vi "Create Gradient Picture.vi"(7 "Border Settings":T1={"Border"=enum."No Border", "Border Color"=10405366, "Border Width"=2, "Oval Width"=15, "Oval Height"=15}, 8 "Offset":cluster{"x":i16, "y":i16}, 9 "Width":i32=50, 10 "Height":i32=200, 11 "Color Array":u32[](array[colorbox])=[9144575, 11917531, 11534591]) -> (3 "Gradient Picture":picture)   [LabVIEW 2016, in "Graphics.lvclass"]
doc: "This VI will draw a gradient picture, which is a 2D picture that is a rectangle at the specified offset, with the height and width provided. Drawing the borders will make the rectangle or rounded rectangle with a border color selected. The gradient goes from the Color Array where index 0 is the top and the last element is the bottom with a gradient between.\n\nhttps://decibel.ni.com/content/docs/DOC-9294\n\n-----\nBrian Hoover (hooovahh)"
uses:
  <resource>/Framework/Providers/Open_GDS/UML/Graphics_class/Graphics.lvclass
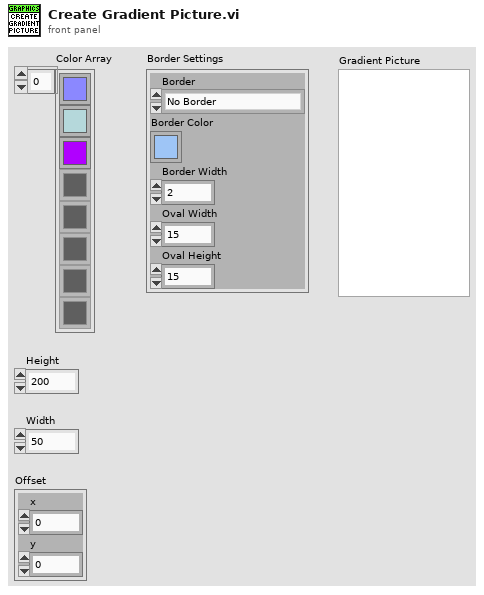
[diagram p1: front panel]
types:
  T1 = cluster{"Border":enum16{"No Border", "Rectangle", "Rounded Rectangle"}, "Border Color":u32, "Border Width":i16, "Oval Width":i16, "Oval Height":i16}
  T2 = enum16{"No Border", "Rectangle", "Rounded Rectangle"}
  T3 = cluster{"left":i16, "top":i16, "right":i16, "bottom":i16}
  T4 = cluster{"Width":i16, "Style":enum32{"Solid", "Dash", "Dot", "DashDot", "DashDotDot"}}
  T5 = cluster{"Width":u16, "Style":enum32{"Solid", "Dash", "Dot", "DashDot", "DashDotDot"}}
  T6 = cluster{"Height":i32, "Width":i32, "Oval Height":i16, "Oval Height":i16, "Border":enum16{"No Border", "Rectangle", "Rounded Rectangle"}, "Border Width":i16, "Border Color":u32}
  T7 = typedef "imagedata.ctl" = cluster{"image type":i32, "image depth":i32, "image":u8[], "mask":u8[], "colors":u32[], "Rectangle":cluster{"left":i16, "top":i16, "right":i16, "bottom":i16}}
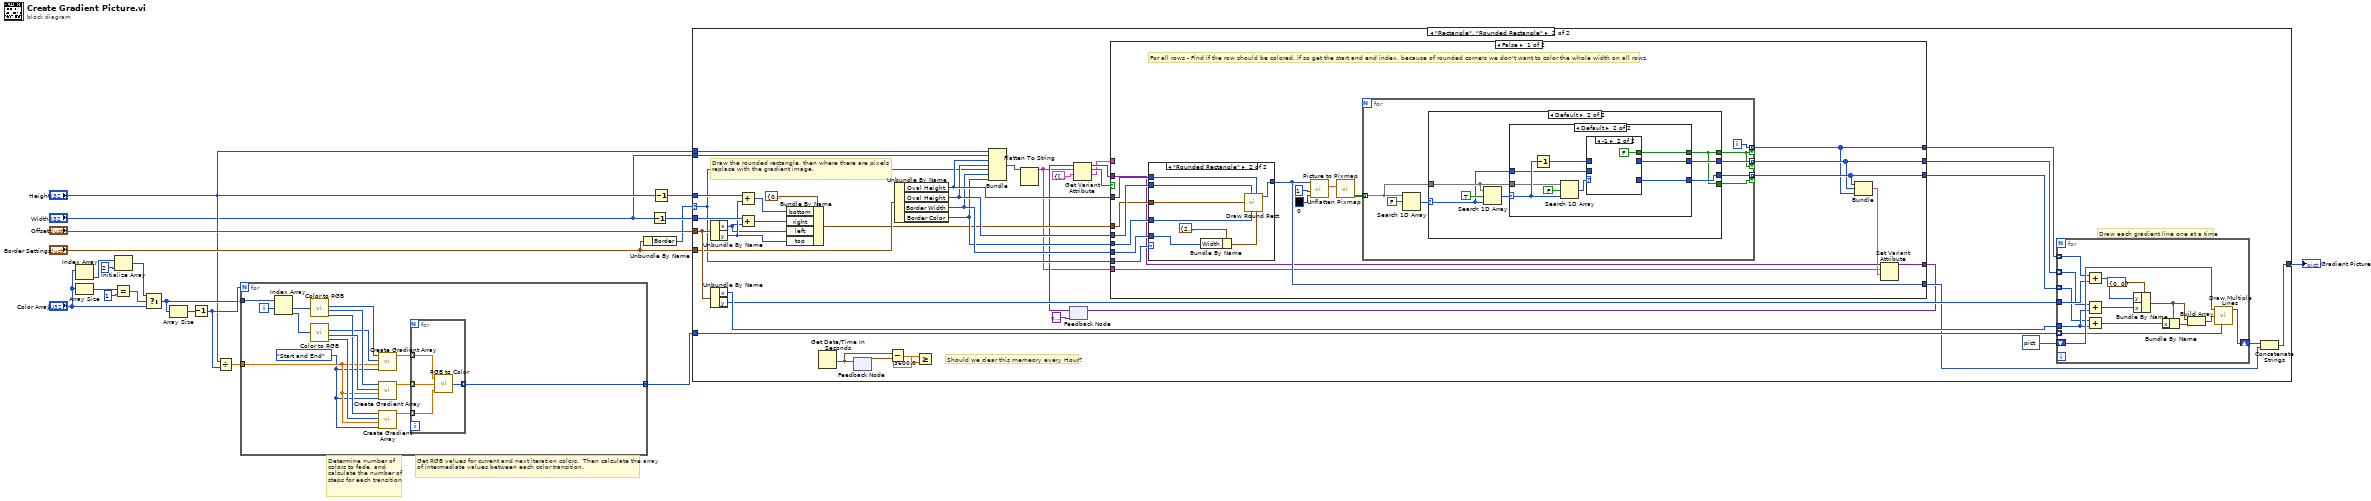
[diagram p0: block diagram]
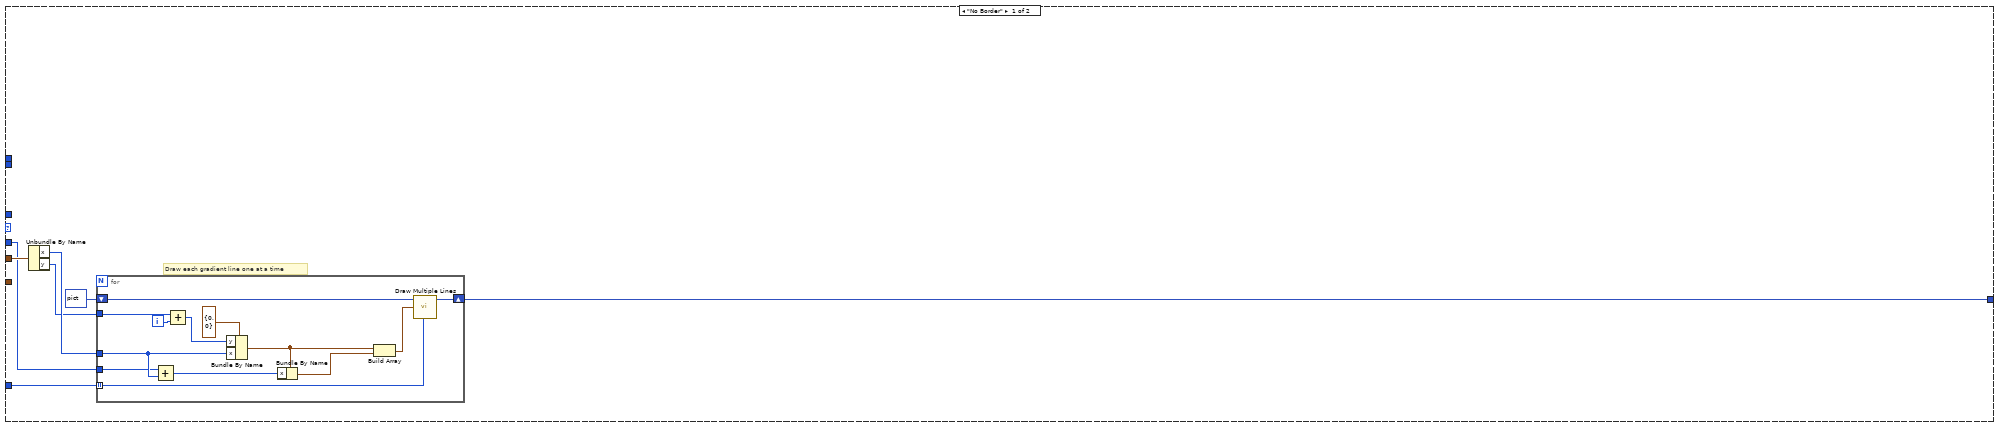
[diagram p2: hidden frame]
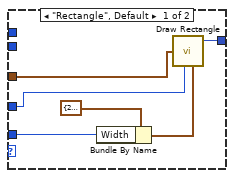
[diagram p3: hidden frame]
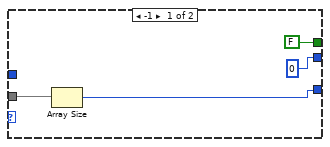
[diagram p5: hidden frame]
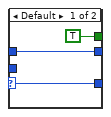
[diagram p6: hidden frame]
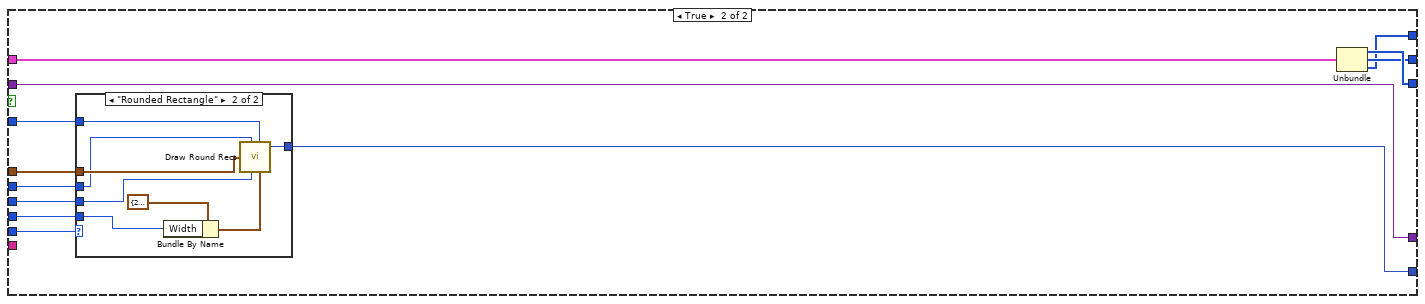
[diagram p7: hidden frame]
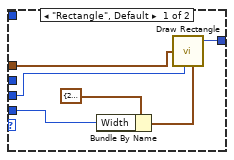
[diagram p8: hidden frame]
diagram:
  # "Get RGB values for current and next iteration colors.  Then calculate the array of intermediate values between each color transition."
  # "Determine number of colors to fade, and calculate the number of steps for each transition"
  n1 = Index Array(array="Color Array") -> (element=w8:u32)  [unwired: 1 in]
  n2 = Array Size(array="Color Array") -> (size(s)=w12:i32)
  n3 = Equal?(x=w12, y=1) -> (x = y?=w10:bool)
  n4 = Initialize Array(w8, 2 ("dimension size")) -> (w6:u32[])
  n5 = Select(t=w6, s=w10, f="Color Array") -> (s? t:f=w5:u32[])
  n6 = Array Size(array=w5) -> (size(s)=w19:i32)
  n7 = Decrement(x=w19) -> (x-1=w18:i32)
  n8 = Divide(x="Height", y=w18) -> (x/y=w20:dbl)
  n9 = for {
    N: w18 -> [_]
    tunnel: w5 -> [w36]
    tunnel: w20 -> [w27]
    tunnel: [w22] -> w17 mode=concatenating
    i -> [w35]
    w26 = enum16{"Start", "End", "Start and End", "None"}."Start and End" ("Values to Include")
    n10 = Index Array(array=w36, index #1=w35) -> (element #1=w34:u32, element #2=w33:u32)  [unwired: 1 in]
    n11 = call <vilib>:"Color to RGB.vi"("Color"=w34) -> ("R"=w32:u8, "G"=w31:u8, "B"=w29:u8)  [unwired: 1 out]
    n12 = call <vilib>:"Color to RGB.vi"("Color"=w33) -> ("R"=w21:u8, "G"=w30:u8, "B"=w28:u8)  [unwired: 1 out]
    n13 = call <resource>:"Create Gradient Array.vi"("Values to Include"=w26, "Array Length"=w27, "End Value"=w21, "Start Value"=w32) -> ("Output Array"=w25:dbl[])  [unwired: 7 in]
    n14 = call <resource>:"Create Gradient Array.vi"("Values to Include"=w26, "Array Length"=w27, "End Value"=w30, "Start Value"=w31) -> ("Output Array"=w24:dbl[])  [unwired: 7 in]
    n15 = call <resource>:"Create Gradient Array.vi"("Values to Include"=w26, "Array Length"=w27, "End Value"=w28, "Start Value"=w29) -> ("Output Array"=w23:dbl[])  [unwired: 7 in]
    n16 = for {
      tunnel: w25 -> [w39] mode=indexing
      tunnel: w24 -> [w40] mode=indexing
      tunnel: w23 -> [w38] mode=indexing
      tunnel: [w37] -> w22 mode=indexing
      n17 = call <vilib>:"RGB to Color.vi"("B"=w38, "G"=w40, "R"=w39) -> ("Color"=w37:u32)
    }
  }
  n18 = Unbundle By Name("Border Settings") -> ("Border"=w3:T2)
  n19 = Decrement(x="Width") -> (x-1=w14:i32)
  n20 = Decrement(x="Height") -> (x-1=w15:i32)
  n21 = case shown="\"Rectangle\", \"Rounded Rectangle\"" w3 {
    selector: w3 -> [_ w80]
    tunnel: [w42 w94] -> w13
    tunnel: w17 -> [w43 w92]
    tunnel: "Offset" -> [w44 w91]
    tunnel: w15 -> [_ w90]
    tunnel: w14 -> [w41 w89]
    tunnel: "Border Settings" -> [_ w83]
    tunnel: "Height" -> [_ w66]
    tunnel: "Width" -> [_ w65]
    frame "No Border" {
      # "Draw each gradient line one at a time"
      n22 = Unbundle By Name(w44) -> ("x"=w46:i16, "y"=w45:i16)
      n23 = for {
        shift-right: [w59] -> w42
        shift-left: picture data[5B] ("picture") -> [w60]
        tunnel: w43 -> [w52] mode=indexing
        tunnel: w45 -> [w51]
        tunnel: w46 -> [w54]
        tunnel: w41 -> [w50]
        i -> [w48]
        n24 = Add(x=w50, y=w54) -> (x+y=w53:i32)
        n25 = Add(x=w51, y=w48) -> (x+y=w49:i32)
        n26 = Bundle By Name(cluster=cluster{"x":i16, "y":i16} {"x"=0, "y"=0} ("point(x,y)"), "y"=w49, "x"=w54) -> (w58:cluster{"x":i16, "y":i16})
        n27 = Bundle By Name(cluster=w58, "x"=w53) -> (w57:cluster{"x":i16, "y":i16})
        n28 = Build Array(w58, w57) -> (w56:cluster{"x":i16, "y":i16}[])
        n29 = call <vilib>:"Draw Multiple Lines.vi"("picture"=w60, "line endpoints"=w56, "color(black)"=w52) -> ("new picture"=w59:picture)  [unwired: 6 in]
      }
    }
    frame "Rectangle", "Rounded Rectangle" {
      # "Should we clear this memeory every Hour?"
      # "Draw each gradient line one at a time"
      # "Draw the rounded rectangle, then where there are pixels replace with the gradient image."
      n30 = Unbundle By Name(w91) -> ("x"=w85:i16, "y"=w87:i16)
      n31 = Unbundle By Name(w91) -> ("x"=w98:i16, "y"=w93:i16)
      n32 = Add(x=w90, y=w87) -> (x+y=w86:i32)
      n33 = Add(x=w89, y=w85) -> (x+y=w84:i32)
      n34 = Bundle By Name(cluster=T3 {"left"=0, "top"=0, "right"=0, "bottom"=0} ("rect"), "bottom"=w86, "right"=w84, "left"=w85, "top"=w87) -> (w77:T3)
      n35 = Get Date/Time In Seconds() -> (seconds since 1Jan1904=w64:timestamp)
      n36 = feedback-in #1(w64) -> ()
      n37 = feedback #1() -> (w63:timestamp)  [unwired: 1 in]
      n38 = Subtract(x=w64, y=w63) -> (x-y=w62:dbl)
      n39 = Unbundle By Name(w83) -> ("Oval Height"=w82:i16, "Oval Height"=w81:i16, "Border Width"=w79:i16, "Border Color"=w78:u32)
      n40 = Greater Or Equal?(x=w62, y=3600.0) -> ()  [unwired: 1 out]
      n41 = Bundle("Height"=w66, "Width"=w65, "Oval Height"=w82, "Oval Height"=w81, "Border"=w80, "Border Width"=w79, "Border Color"=w78) -> (w74:T6)  [unwired: 1 in]
      n42 = Flatten To String(anything=w74) -> (data string=w70:string)  [unwired: 3 in, 2 out]
      n43 = feedback #2(variant ("duplicate variant")) -> (w76:variant)
      n44 = Get Variant Attribute(Variant=w76, name=w70, default value (empty Variant)=cluster{i32[], i32[], i32[]} {[], [], []} ("output cluster")) -> (duplicate Variant=w71:variant, found=w72:bool, value=w67:cluster{i32[], i32[], i32[]})  [unwired: 1 in, 1 out]
      n45 = case shown="False" w72 {
        tunnel: [w106 w172] -> w99
        tunnel: [w107 w173] -> w97
        tunnel: [w108 w174] -> w96
        tunnel: w82 -> [w117 w167]
        tunnel: w81 -> [w116 w166]
        tunnel: w80 -> [w115 w171]
        tunnel: w79 -> [w114 w169]
        tunnel: w78 -> [w113 w168]
        tunnel: w77 -> [w112 w170]
        tunnel: [w105 w165] -> w75
        tunnel: w71 -> [w104 w176]
        tunnel: w70 -> [w102 _]
        tunnel: [w101 w176] -> w69
        tunnel: w67 -> [_ w175]
        frame False {
          # "For all rows - Find if the row should be colored, if so get the start and end index, because of rounded corners we don't want to color the whole width on all rows."
          n46 = case shown="\"Rounded Rectangle\"" w115 {
            tunnel: w113 -> [w123 w129]
            tunnel: [w122 w132] -> w105
            tunnel: w112 -> [w124 w130]
            tunnel: w114 -> [w119 w127]
            tunnel: w117 -> [_ w126]
            tunnel: w116 -> [_ w125]
            frame "Rectangle", Default {
              n47 = Bundle By Name(cluster=T4 {"Width"=2, "Style"=enum."Solid"} ("pen"), "Width"=w119) -> (w120:T4)
              n48 = call <vilib>:"Draw Rectangle.vi"("rect"=w124, "color(black)"=w123, "pen"=w120) -> ("new picture"=w122:picture)  [unwired: 6 in]
            }
            frame "Rounded Rectangle" {
              n49 = Bundle By Name(cluster=T5 {"Width"=2, "Style"=enum."Solid"} ("pen"), "Width"=w127) -> (w128:T5)
              n50 = call <vilib>:"Draw Round Rect.vi"("oval width"=w125, "rect"=w130, "color(black)"=w129, "oval height"=w126, "pen"=w128) -> ("new picture"=w132:picture)  [unwired: 4 in]
            }
          }
          n51 = call <vilib>:"Picture to Pixmap.vi"("Background Color"=u32 0, "depth"=1, "picture"=w105) -> ("image data"=w110:T7)  [unwired: 7 in, 1 out]
          n52 = call <vilib>:"Unflatten Pixmap.vi"("image data"=w110) -> ("1-bit pixmap"=w118:bool[][])  [unwired: 4 in, 6 out]
          n53 = for {
            tunnel: w118 -> [w139] mode=indexing
            tunnel: [w137] -> w107 mode=indexing if=w133
            tunnel: [w136] -> w108 mode=indexing if=w135
            tunnel: [w134] -> w106 mode=indexing if=w133
            i -> [w134]
            n54 = Search 1D Array(1D array=w139, element=FALSE) -> (index of element=w138:i32)  [unwired: 1 in]
            n55 = case shown="Default" w138 {
              selector: w138 -> [_ w143]
              tunnel: w139 -> [_ w145]
              tunnel: [_ w142] -> w137
              tunnel: [_ w144] -> w136
              tunnel: [_ w141] -> w135
              tunnel: [_ w141] -> w133
              frame -1 {
              }
              frame Default {
                n56 = Search 1D Array(1D array=w145, element=TRUE, start index (0)=w143) -> (index of element=w146:i32)
                n57 = case shown="Default" w146 {
                  selector: w146 -> [_ w159]
                  tunnel: w145 -> [w151 w153]
                  tunnel: [w150 w154] -> w144
                  tunnel: w143 -> [_ w156]
                  tunnel: [0 ("index of element") w155] -> w142
                  tunnel: [FALSE w152] -> w141
                  frame -1 {
                    n58 = Array Size(array=w151) -> (size(s)=w150:i32)
                  }
                  frame Default {
                    n59 = Decrement(x=w159) -> (x-1=w157:i32)
                    n60 = Search 1D Array(1D array=w153, element=FALSE, start index (0)=w159) -> (index of element=w158:i32)
                    n61 = case shown="-1" w158 {
                      selector: w158 -> [w162 _]
                      tunnel: w157 -> [w163 _]
                      tunnel: w156 -> [_ _]
                      tunnel: [w163 _] -> w155
                      tunnel: [w162 _] -> w154
                      tunnel: [TRUE FALSE] -> w152
                      frame Default {
                      }
                      frame -1 {
                      }
                    }
                  }
                }
              }
            }
          }
          n62 = Bundle(w108, w107, w106) -> (w103:cluster{i32[], i32[], i32[]})  [unwired: 1 in]
          n63 = Set Variant Attribute(Variant=w104, name=w102, value=w103) -> (Variant out=w101:variant)  [unwired: 1 in, 2 out]
        }
        frame True {
          n64 = case shown="\"Rounded Rectangle\"" w171 {
            tunnel: w168 -> [w181 w187]
            tunnel: [w180 w190] -> w165
            tunnel: w170 -> [w182 w188]
            tunnel: w169 -> [w177 w185]
            tunnel: w167 -> [_ w184]
            tunnel: w166 -> [_ w183]
            frame "Rectangle", Default {
              n65 = Bundle By Name(cluster=T4 {"Width"=2, "Style"=enum."Solid"} ("pen"), "Width"=w177) -> (w178:T4)
              n66 = call <vilib>:"Draw Rectangle.vi"("rect"=w182, "color(black)"=w181, "pen"=w178) -> ("new picture"=w180:picture)  [unwired: 6 in]
            }
            frame "Rounded Rectangle" {
              n67 = Bundle By Name(cluster=T5 {"Width"=2, "Style"=enum."Solid"} ("pen"), "Width"=w185) -> (w186:T5)
              n68 = call <vilib>:"Draw Round Rect.vi"("oval width"=w183, "rect"=w188, "color(black)"=w187, "oval height"=w184, "pen"=w186) -> ("new picture"=w190:picture)  [unwired: 4 in]
            }
          }
          n69 = Unbundle(w175) -> (w174:i32[], w173:i32[], w172:i32[])
        }
      }
      n70 = feedback-in #2(w69) -> ()
      n71 = for {
        shift-right: [w204] -> w95
        shift-left: picture data[5B] ("picture") -> [w205]
        tunnel: w92 -> [w191] mode=indexing
        tunnel: w99 -> [w200] mode=indexing
        tunnel: w93 -> [w199]
        tunnel: w98 -> [w194]
        tunnel: w97 -> [w195] mode=indexing
        tunnel: w96 -> [w193] mode=indexing
        n72 = Add(x=w200, y=w199) -> (x+y=w198:i32)
        n73 = Add(x=w195, y=w194) -> (x+y=w196:i32)
        n74 = Add(x=w193, y=w194) -> (x+y=w192:i32)
        n75 = Bundle By Name(cluster=cluster{"x":i16, "y":i16} {"x"=0, "y"=0} ("point(x,y)"), "y"=w198, "x"=w196) -> (w203:cluster{"x":i16, "y":i16})
        n76 = Bundle By Name(cluster=w203, "x"=w192) -> (w202:cluster{"x":i16, "y":i16})
        n77 = Build Array(w203, w202) -> (w201:cluster{"x":i16, "y":i16}[])
        n78 = call <vilib>:"Draw Multiple Lines.vi"("picture"=w205, "line endpoints"=w201, "color(black)"=w191) -> ("new picture"=w204:picture)  [unwired: 6 in]
      }
      n79 = Concatenate Strings(w95, w75) -> (w94:picture)
    }
  }
  "Gradient Picture" <- w13
